vi "SR830-sensitivity.vi"(8 "error in (no error)":errorcluster, 10 "Sensitivity (-1: Auto gain)":i16(ring)=-1 items=["Auto Gain"=-1, "2 nV/fA"=0, "5 nV/fA"=1, "10 nV/fA"=2, "20 nV/fA"=3, "50 nV/fA"=4, "100 nV/fA"=5, "200 nV/fA"=6, "500 nV/fA"=7, "1 uV/pA"=8, "2 uV/pA"=9, "5 uV/pA"=10, "10 uV/pA"=11, "20 uV/pA"=12, "50 uV/pA"=13, "100 uV/pA"=14, "200 uV/pA"=15, "500 uV/pA"=16, "1 mV/nA"=17, "2 mV/nA"=18, "5 mV/nA"=19, "10 mV/nA"=20, "20 mV/nA"=21, "50 mV/nA"=22, "100 mV/nA"=23, "200 mV/nA"=24, "500 mV/mA"=25, "1 V/uA"=26], 11 "VISA resource name":refnum<visa-resource-name>) -> (0 "error out":errorcluster, 3 "VISA resource name out":refnum<visa-resource-name>)   [LabVIEW 2019, in "SubVI.lvlib"]
uses:
  SubVI.lvlib
  lib/Stanford Research 830/Stanford Research 830.lvlib
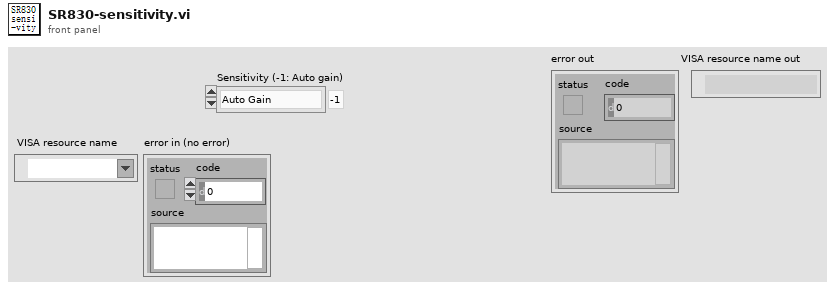
[diagram p1: front panel]
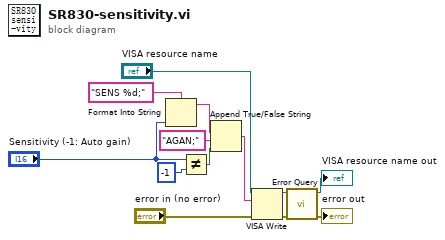
[diagram p0: block diagram]
diagram:
  n1 = Format Into String(format string="SENS %d;", "Sensitivity (-1: Auto gain)") -> (resulting string=w3:string)  [unwired: 2 in, 1 out]
  n2 = Not Equal?(x="Sensitivity (-1: Auto gain)", y=i16 -1) -> (x != y?=w4:bool)
  n3 = Append True/False String(1:w4, 2:"AGAN;" ("false string"), 3:w3) -> (0:w1:string)  [unwired: 1 in]
  n4 = VISA Write(VISA resource name="VISA resource name", write buffer=w1, error in (no error)="error in (no error)") -> (VISA resource name out=w13:refnum<visa-resource-name>, error out=w9:errorcluster)  [unwired: 1 out]
  n5 = call "Error Query.vi"("error in (no error)"=w9, "VISA resource name"=w13) -> ("error out"=→"error out":errorcluster, "VISA resource name out"=→"VISA resource name out":refnum<visa-resource-name>)  [unwired: 7 in, 1 out]
